vi "Build Servo Hello.vi"(11 "Familiar":bool) -> (3 "String":string)   [LabVIEW 2017]
uses:
  <vilib>/Rock Robotics/Network Tables/NT Globals.vi
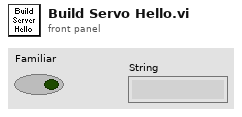
[diagram p1: front panel]
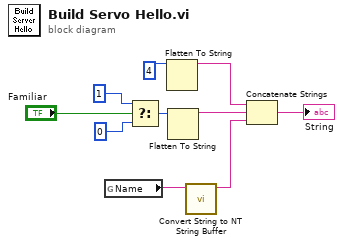
[diagram p0: block diagram]
diagram:
  n1 = global read "NT Globals.vi" "Name"() -> (w7:string)
  n2 = Select(t=u8 1 ("bytes to read"), s="Familiar", f=u8 0 ("bytes to read")) -> (s? t:f=w4:u8)
  n3 = Flatten To String(anything=u8 4 ("bytes to read")) -> (data string=w9:string)  [unwired: 3 in, 2 out]
  n4 = Flatten To String(anything=w4) -> (data string=w5:string)  [unwired: 3 in, 2 out]
  n5 = call <vilib>:"Convert String to NT String Buffer.vi"("LV Buffer"=w7) -> ("NT Buffer"=w6:string)  [unwired: 10 in]
  n6 = Concatenate Strings(w9, w5, w6) -> (→"String":string)
